vi "SubVI_RampSpeedDown_Teleop.vi"() -> ()   [LabVIEW 2017]
panel:
  in  "Y Axis Input(Changing Value)":dbl
  out "Y Axis Output":dbl
  in  "Number Of Iterations":i32=7
  in  "Y Axis Input(Not Changing)":dbl
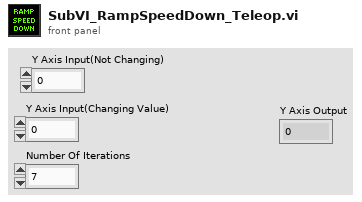
[diagram p1: front panel]
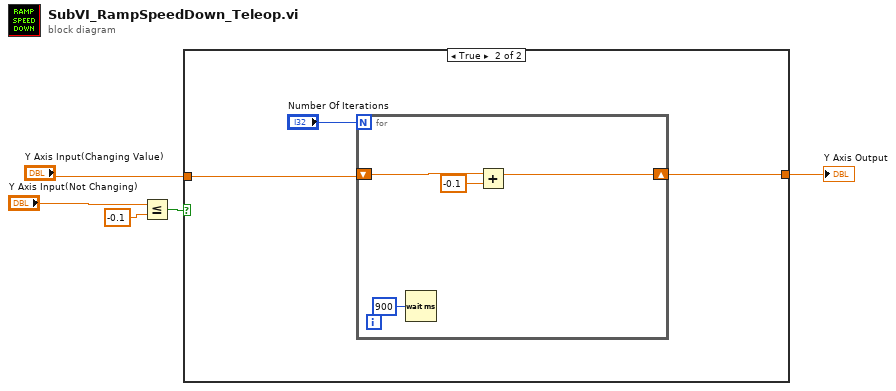
[diagram p0: block diagram]
diagram:
  n1 = Less Or Equal?(x="Y Axis Input(Not Changing)", y=-0.1) -> (x <= y?=w3:bool)
  n2 = case shown="True" w3 {
    tunnel: [w6 w7] -> w2
    tunnel: "Y Axis Input(Changing Value)" -> [w6 w8]
    frame False {
    }
    frame True {
      n3 = for {
        N: "Number Of Iterations" -> [_]
        shift-right: [w10] -> w7
        shift-left: w8 -> [w12]
        n4 = Wait (ms)(milliseconds to wait=u32 900) -> ()  [unwired: 1 out]
        n5 = Add(x=w12, y=-0.1) -> (x+y=w10:dbl)
      }
    }
  }
  "Y Axis Output" <- w2
